vi "Rename Plugin Data File.vi"(0 "configuration":T1, 5 "Plugin Library Path":path, 11 "error in":errorcluster) -> (4 "Plugin Data File Path":path, 15 "error out":errorcluster)   [LabVIEW 2021, in "InstrumentStudio Plug-In Editor.lvlib"]
uses:
  InstrumentStudio Plug-In Editor.lvlib
  controls/Data Holder.ctl
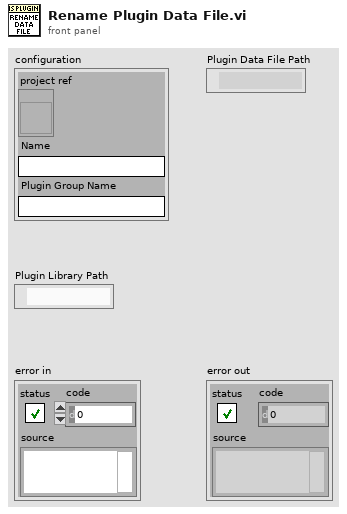
[diagram p1: front panel]
types:
  T1 = typedef "InstrumentStudio Plug-In Editor.lvlib/Data Holder.ctl" = cluster{"project ref":refnum<vi>, "Name":string, "Plugin Group Name":string}
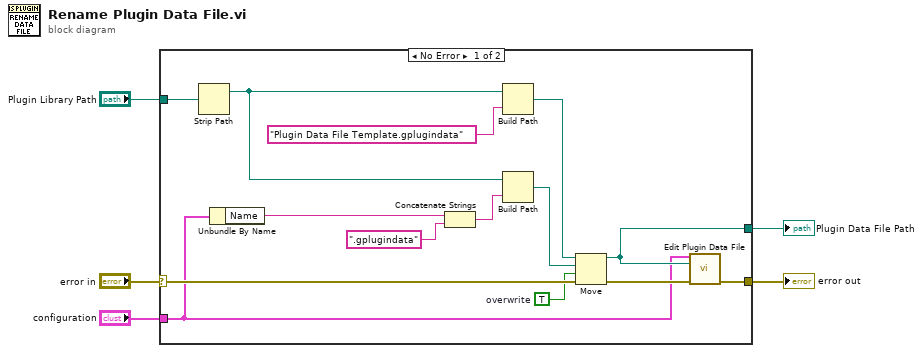
[diagram p0: block diagram]
diagram:
  n1 = case shown="No Error" "error in" {
    selector: "error in" -> [w19 w20]
    tunnel: [w17 w20] -> w5
    tunnel: "configuration" -> [w11 _]
    tunnel: [w12 _] -> w4
    tunnel: "Plugin Library Path" -> [w8 _]
    frame No Error {
      w13 = TRUE  # overwrite
      n2 = Strip Path(path=w8) -> (stripped path=w6:path)  [unwired: 1 out]
      n3 = Unbundle By Name(w11) -> ("Name"=w16:string)
      n4 = Concatenate Strings(w16, ".gplugindata" ("string")) -> (w7:string)
      n5 = Build Path(base path=w6, name or relative path="Plugin Data File Template.gplugindata" ("string")) -> (appended path=w15:path)
      n6 = Build Path(base path=w6, name or relative path=w7) -> (appended path=w14:path)
      n7 = Move(source path=w15, error in=w19, 9:w13, 10:w14) -> (error out=w18:errorcluster, 3:w12:path)  [unwired: 1 in, 1 out]
      n8 = call "Edit Plugin Data File.vi"("configuration"=w11, "Data File Path"=w12, "error in"=w18) -> ("error out"=w17:errorcluster)  [unwired: 12 in]
    }
    frame Error {
    }
  }
  "error out" <- w5
  "Plugin Data File Path" <- w4
